vi "cRIO - Check Time Sync.vi"(8 "Error In":errorcluster, 9 "Time Sync Tolerance (60sec)":dbl=60.0 format="%#_13g", 10 "Timeout (minutes)":i32=5, 11 "cRIO Timestamp SV":string="ni.var.psp://192.168.1.50/RT Library/cRIO Timestamp") -> (0 "error out 4":errorcluster, 1 "seconds waited":dbl format="%.1f", 2 "cRIO Timestamp SYNCed":bool, 3 "cRIO Timestamp":timestamp)   [LabVIEW 2013]
uses:
  <resource>/objmgr/ni.var.rc
panel:
  out "Local Time":timestamp
  out "error out 3":errorcluster
  out "error out 2":errorcluster
  out "error out":errorcluster
  out "Readable":bool
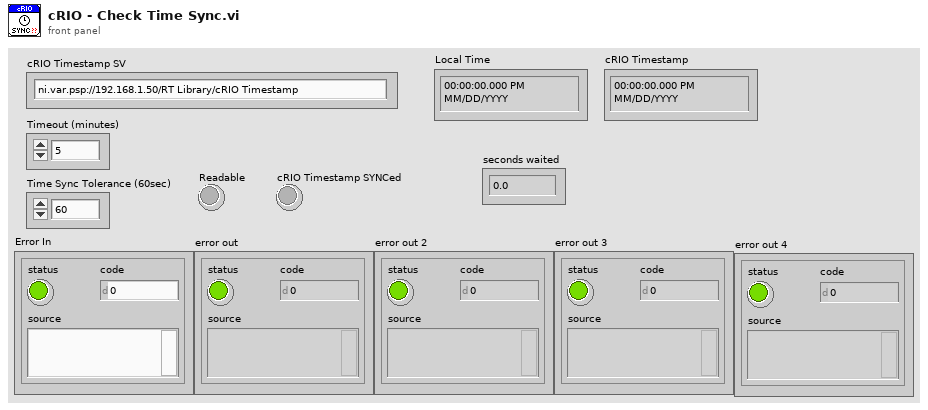
[diagram p1: front panel]
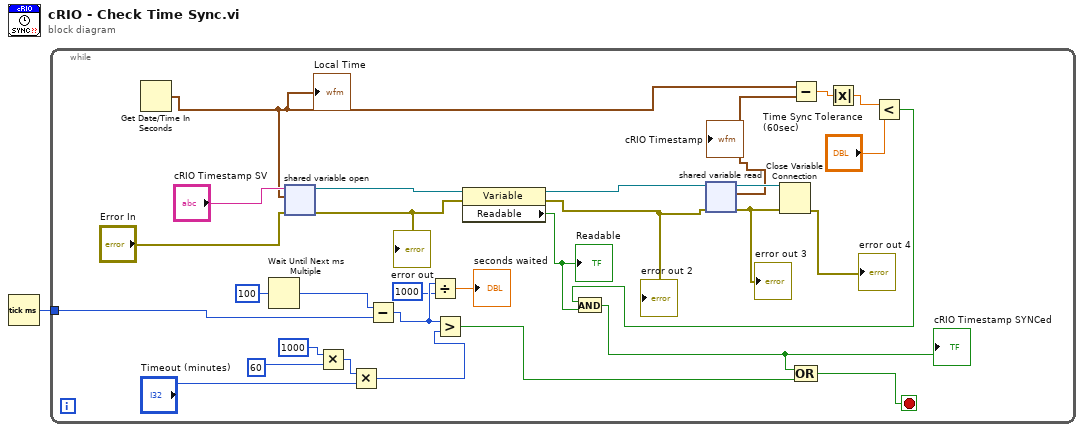
[diagram p0: block diagram]
diagram:
  n1 = Tick Count (ms)() -> (millisecond timer value=w1:u32)
  n2 = while {
    tunnel: w1 -> [w23]
    stop <- w16 stop-if-true
    n3 = Get Date/Time In Seconds() -> (seconds since 1Jan1904=w9:timestamp)
    "Local Time" <- w9
    n4 = Wait Until Next ms Multiple(millisecond multiple=u32 100) -> (millisecond timer value=w24:u32)
    n5 = shared-variable-open("cRIO Timestamp SV", "Error In", w9) -> (w30:refnum<k21>, w29:errorcluster)  [unwired: 1 in]
    "error out" <- w29
    n6 = Multiply(x=1000, y=60) -> (x*y=w20:i32)
    n7 = Multiply(x=w20, y="Timeout (minutes)") -> (x*y=w18:i32)
    n8 = Subtract(x=w24, y=w23) -> (x-y=w15:u32)
    n9 = Divide(x=w15, y=1000) -> (x/y=→"seconds waited":dbl)
    n10 = Greater?(x=w15, y=w18) -> (0:w17:bool)
    n11 = property class="Variable"(reference=w30, error in=w29) -> (reference out=w28:refnum<k21>, error out=w27:errorcluster, "Readable"=w7:bool)
    "Readable" <- w7
    "error out 2" <- w27
    n12 = shared-variable-read(w28, w27) -> (w26:refnum<k21>, w4:errorcluster, w8:timestamp)  [unwired: 1 out]
    "error out 3" <- w4
    "cRIO Timestamp" <- w8
    n13 = Close Variable Connection(8:w4, 11:w26) -> (0:→"error out 4":errorcluster)
    n14 = Subtract(x=w9, y=w8) -> (x-y=w12:dbl)
    n15 = Absolute Value(x=w12) -> (abs(x)=w11:dbl)
    n16 = Less?(x=w11, y="Time Sync Tolerance (60sec)") -> (x < y?=w6:bool)
    n17 = And(x=w6, y=w7) -> (x .and. y?=w5:bool)
    "cRIO Timestamp SYNCed" <- w5
    n18 = Compound Arithmetic op=OR(w5, w17) -> (w16:bool)
  }
